vi "Noise BW from IIR Cluster.vi"(9 "samples":i32=10000, 10 "IIR Filter Cluster":T1) -> (3 "noise bandwidth":dbl=1.0)   [LabVIEW 2017, in "NI_AALBase.lvlib"]
uses:
  NI_AALBase.lvlib
  IIR Cascade Filter (DBL).vi
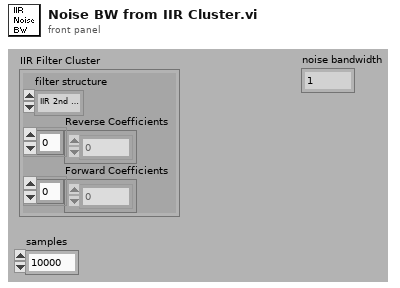
[diagram p1: front panel]
types:
  T1 = cluster{"filter structure":enum32{"IIR 2nd Order", "IIR 4th Order"}, "Reverse Coefficients":dbl[], "Forward Coefficients":dbl[]}
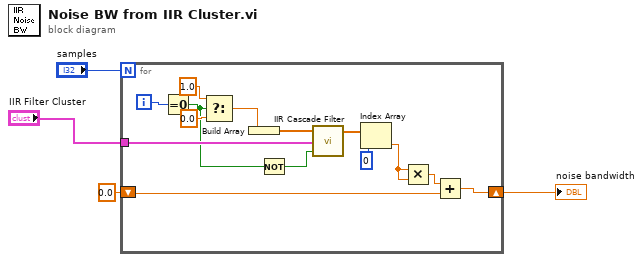
[diagram p0: block diagram]
diagram:
  n1 = for {
    N: "samples" -> [_]
    tunnel: "IIR Filter Cluster" -> [w18]
    shift-right: [w8] -> w1
    shift-left: 0.0 -> [w11]
    i -> [w17]
    n2 = Equal To 0?(x=w17) -> (x = 0?=w5:bool)
    n3 = Select(t=1.0, s=w5, f=0.0) -> (s? t:f=w14:dbl)
    n4 = Build Array(w14) -> (w13:dbl[])
    n5 = Not(x=w5) -> (.not. x?=w6:bool)
    n6 = call-poly "IIR Cascade Filter.vi"("init/cont (init:F)"=w6, "IIR Filter Cluster"=w18, "X"=w13) -> ("Filtered X"=w12:dbl[])  [unwired: 1 out]
    n7 = Index Array(array=w12, index=0) -> (element=w10:dbl)
    n8 = Multiply(x=w10, y=w10) -> (x*y=w7:dbl)
    n9 = Add(x=w7, y=w11) -> (x+y=w8:dbl)
  }
  "noise bandwidth" <- w1
